vi "Connect.vi"(8 "error in":errorcluster, 11 "69X_79X in":refnum<class "6972A.lvclass">) -> (0 "error out":errorcluster, 3 "69X_79X out":refnum<class "6972A.lvclass">)   [LabVIEW 2019, in "6972A.lvlib" / "6972A.lvclass"]
uses:
  Library/6972A.lvclass
  C:/Users/Public/Documents/Development/builds/Instruments/Instruments.lvlibp/Library/Instruments.lvclass
  Library/6972A.lvclass/6972A.ctl
  builds/Instruments/Instruments.lvlibp/Accessors/Read Resource.vi
  <instrlib>/Agilent N6900 N7900 Series/Agilent N6900 N7900 Series.lvlib
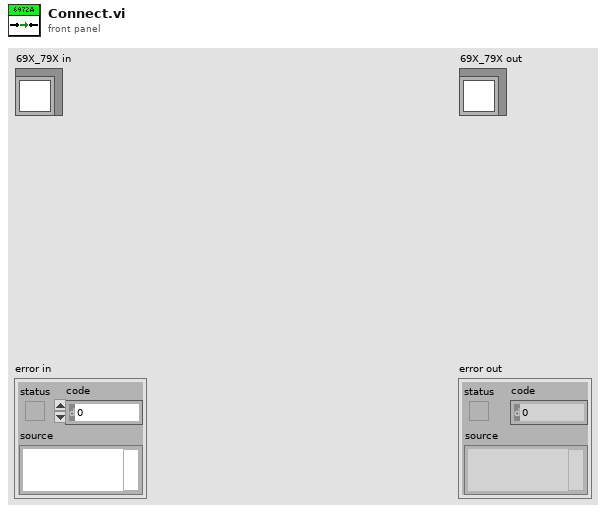
[diagram p1: front panel]
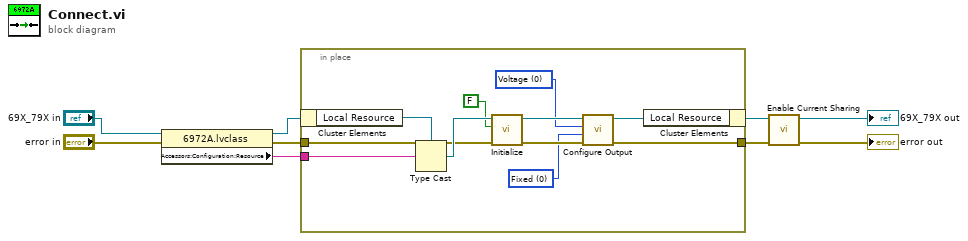
[diagram p0: block diagram]
diagram:
  n1 = property class="6972A.lvclass"(reference="69X_79X in", error in="error in") -> (reference out=w4:refnum<class "6972A.lvclass">, error out=w3:errorcluster, "Accessors:Configuration:Resource"=w5:string)
  n2 = in-place {
    in-place-border: w5 -> [w19]
    in-place-border: w3 -> [w17]
    in-place-border: [w12] -> w9
    w10 = u16 0 items=["Fixed", "Step", "List", "Arbitrary"] ("Output Transient Mode (0: Fixed)")
    w11 = u16 0 items=["Voltage", "Current"] ("Output Priority Mode (0: Voltage)")
    n3 = in-place-cluster #1(w4) -> ("Local Resource"=w20:refnum<visa-resource-name>)
    n4 = Type Cast(type=w20, x=w19) -> (*(type *) &x=w18:refnum<visa-resource-name>)
    n5 = call <instrlib>:"Initialize.vi"("error in (no error)"=w17, "ID Query (True)"=FALSE, "VISA resource name"=w18) -> ("error out"=w13:errorcluster, "VISA resource name out"=w15:refnum<visa-resource-name>)  [unwired: 7 in]
    n6 = call <instrlib>:"Configure Output.vi"("error in (no error)"=w13, "Output Transient Mode (0: Fixed)"=w10, "Output Priority Mode (0: Voltage)"=w11, "VISA resource name"=w15) -> ("error out"=w12:errorcluster, "VISA resource name out"=w14:refnum<visa-resource-name>)  [unwired: 6 in]
    n7 = in-place-cluster #1("Local Resource"=w14) -> (w8:refnum<class "6972A.lvclass">)
  }
  n8 = call "Enable Current Sharing.vi"("error in (no error)"=w9, "69X_79X in"=w8) -> ("error out"=→"error out":errorcluster, "69X_79X out"=→"69X_79X out":refnum<class "6972A.lvclass">)  [unwired: 8 in]
